vi "Firmware.vi"() -> ()   [LabVIEW 2017]
uses:
  <vilib>/Platform/TimedLoop/XDataNode/timing_clust.ctl
  <vilib>/Platform/TimedLoop/XDataNode/nitl_modes.ctl
  <vilib>/Platform/TimedLoop/XDataNode/wakeup.ctl
  modInput.ctl
  <instrlib>/_niInstr/Instruction Framework/v1/FPGA/Helper Classes/Single Address Space Collection/Single Address Space Collection.lvclass
  C:/Program Files (x86)/National Instruments/LabVIEW 2017/instr.lib/_niInstr/Instruction Framework/v1/FPGA/Interfaces/Address Space Collection/Address Space Collection.lvclass
  <instrlib>/_niInstr/FIFO Register Bus/v1/FPGA/niInstr FIFO Register Bus v1 FPGA.lvclass
  C:/Program Files (x86)/National Instruments/LabVIEW 2017/instr.lib/_niInstr/Instruction Framework/v1/FPGA/Interfaces/Instruction Producer/Instruction Producer.lvclass
  <vilib>/rvi/Emulation/niFpgaGetClockAttributes.vi
  <vilib>/rvi/Emulation/niFpgaSctlEmulationGetInTimedLoop.vi
  <vilib>/rvi/Emulation/niFpgaEmulationReportErrorSimple.vi
  <vilib>/rvi/Emulation/niFpgaProcessEmulError.vi
  <vilib>/rvi/Emulation/niFpgaCriticalErrorInLSC.vi
  <vilib>/rvi/eio/common/nirviEmuTemplateMethod_errors.vi
  <vilib>/eio/EIONode/EIONode.xnode
  <vilib>/Platform/TimedLoop/XDataNode/XDataNode.xnode
  <instrlib>/_niInstr/Instruction Framework/v1/FPGA/Top Level Bus/Register Configuration/Register Configuration.lvclass
  <vilib>/Platform/TimedLoop/XDataNode/XDNodeRunTimeDep.lvlib
  <vilib>/NI/PowerElectronicsControl/ScaleAndLimit/Core/ScaleAndLimit.lvlib
  <vilib>/NI/PowerElectronicsControl/ScaleAndLimit/Core/AddressSpace.lvclass
  <vilib>/NI/PowerElectronicsControl/WaveformAcq/FPGA/WaveformAddressSpace.lvclass
  BuckBoost.lvlib
  AddressSpace.lvclass
panel:
  out "errors":sgl[](array[numeric])
  out "I_BuckBoost":sgl[](array[numeric])
  out "perturbance":sgl
  in  "desiredSimultaneousAILoopRate":u32 caption="Count(Ticks)"
  out "actualBuckBoostRate":u32
  in  "desiredBuckBoostRate":u32
  out "signal":fxp<+,18,0>[](array[numeric])
  in  "I_setpt":sgl format="%#_13g"
  in  "ManualTrigger":bool
  out "TriggerTimestamp":i32
  out "FaultBuffer":u64 format="%.0x"
  out "relativeTimestamp":i32
  in  "fifo reg bus ctrl 0":u32
  out "fifo reg bus status 0":u32
  out "fifo reg bus data 0":u64
  out "actualSimultaneousAILoopRate":u32
  out "LimitsFlag":bool
  out "Simultaneous_AI":sgl[](array[numeric])
  # "Device Utilization\n---------------------------\nTotal Slices: 66.8% (8878 out of 13300)\nSlice Registers: 25.5% (27136 out of 106400)\nSlice LUTs: 44.1% (23463 out of 53200)\nBlock RAMs: 5.0% (7 out of 140)\nDSP48s: 1.8% (4 out of 220)"
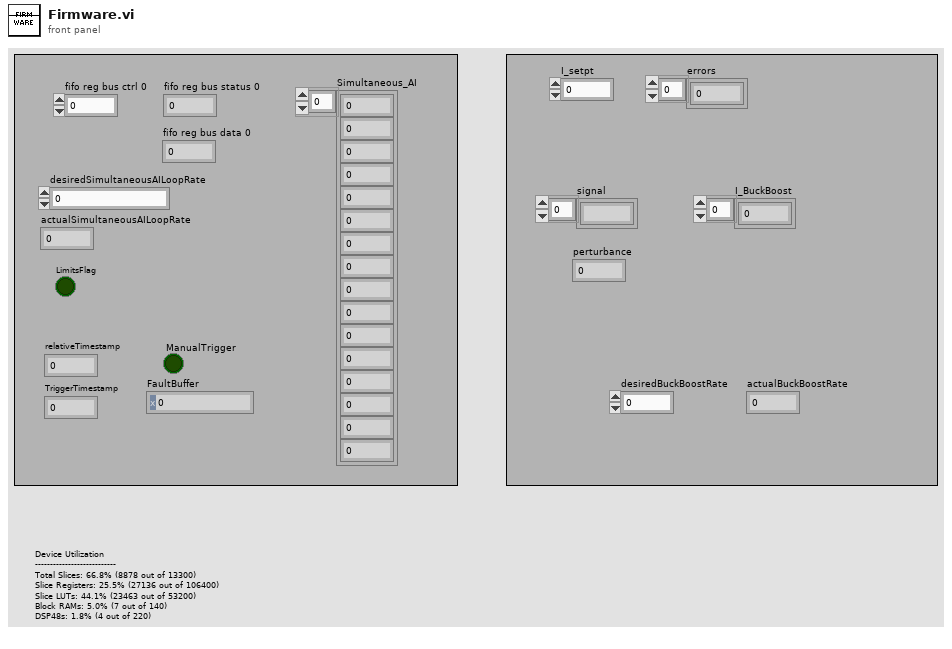
[diagram p1: front panel]
types:
  T1 = typedef "BuckBoost.lvlib/contSettings.ctl" = cluster{"numberOfInterleaves":refnum<k21>, "rampRate":refnum<k21>, "manualInput":refnum<k21>, "perturbAmp":refnum<k21>, "perturbAngleInc":refnum<k21>, "reset":refnum<k21>, "state":refnum<k21>, "gains":refnum<k21>, "Currents":refnum<k21>}
  T2 = typedef "BuckBoost.lvlib/modRegisters.ctl" = cluster{"numberOfInterleaves":refnum<k21>, "Enable":refnum<k21>, "triangleInc":refnum<k21>, "Deadband":refnum<k21>, "Enabled":refnum<k21>}
  T3 = typedef "XDNodeRunTimeDep.lvlib/timing_clust.ctl" = cluster{"Expected End [f-1]":u64, "Actual End [f-1]":u64, "Finished Late? [f-1]":bool, "Expected End [i-1]":u64, "Actual End [i-1]":u64, "Finished Late? [i-1]":bool, "Expected Start [i]":u64, "Actual Start [i]":u64, "Expected Start [f]":u64, "Actual Start [f]":u64, "Source Name":string, "Structure Name":string, "Period":i64, "Deadline":i64, "Offset":i64, "Start":i64, "Priority":i32, "Timeout":i32, "Mode":T4, "Wakeup Reason":T5, "Error":errorcluster, "Source Type":string, "Secondary Source Type":string, "Global End Time":u64, "Global Start Time":u64, "Frame Duration":u64, "Iteration Duration":u64, "Assigned CPU":i32, "I/O Scan Engine Mode":u32}
  T4 = typedef "XDNodeRunTimeDep.lvlib/nitl_modes.ctl" = enum32{"No Change", "Process missed periods, maintain original phase", "Discard missed periods, maintain original phase", "Process missed periods, ignore original phase", "Discard missed periods, ignore original phase"}
  T5 = typedef "XDNodeRunTimeDep.lvlib/wakeup.ctl" = enum32{"Normal", "Aborted", "Asynchronous wakeup", "Timing source error", "Timed loop error", "Timeout"}
  T6 = typedef "BuckBoost.lvlib/modInput.ctl" = cluster{"signal":fxp<+,18,0>[]}
  T7 = typedef "BuckBoost.lvlib/modOutput.ctl" = cluster{"Top":bool, "Bottom":bool}
  T8 = typedef "ScaleAndLimit.lvlib/LimitsRegisters.ctl" = cluster{"HighLimits":refnum<k21>, "LowLimits":refnum<k21>, "ClearLimits":refnum<k21>, "LimitsFlag":refnum<k21>}
  T9 = typedef "ScaleAndLimit.lvlib/ConfigRegisters.ctl" = cluster{"LimitsEnabled":refnum<k21>, "UnscaledHighLimit":refnum<k21>, "UnscaledLowLimit":refnum<k21>, "B":refnum<k21>, "M":refnum<k21>}
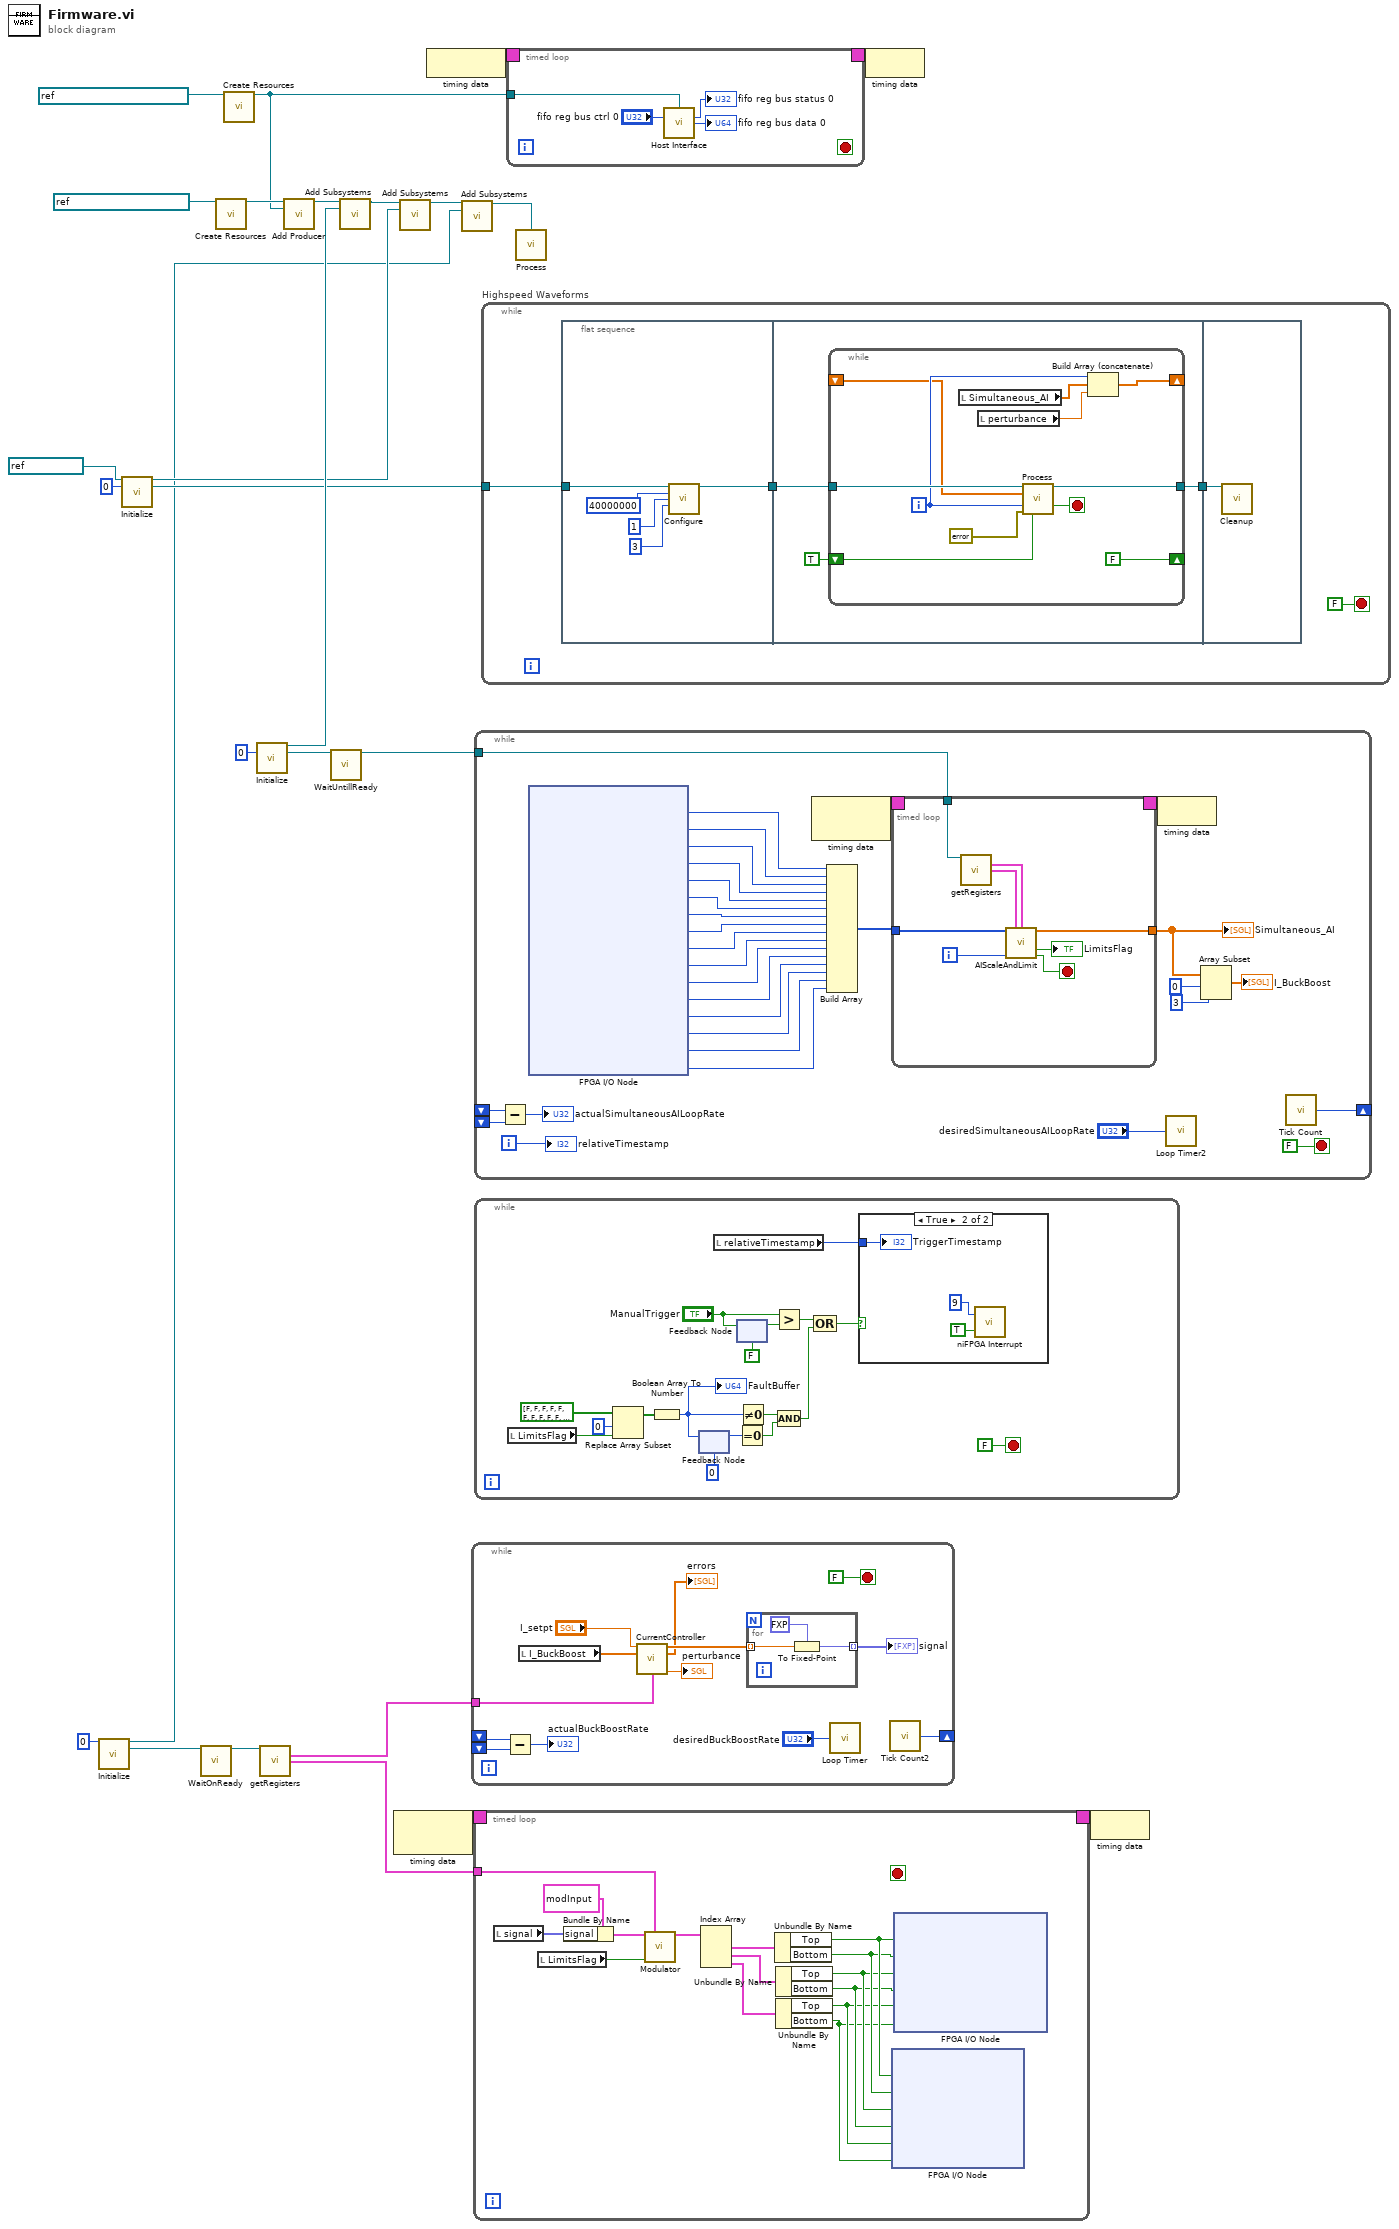
[diagram p0: block diagram]
diagram:
  n1 = call <vilib>:"Initialize.vi"("instance"=u8 0) -> ("subsystem"=w9:refnum<class "Single Address Space Collection.lvclass">, "AddressSpace"=w6:refnum<class "AddressSpace.lvclass">)  [unwired: 13 in]
  n2 = call <vilib>:"Initialize.vi"("DMA FIFO"=refnum<k21> "DataSGL0" ("FIFO Out"), "instance"=u8 0) -> ("subsystem"=w12:refnum<class "Single Address Space Collection.lvclass">, "AddressSpace"=w15:refnum<class "WaveformAddressSpace.lvclass">)  [unwired: 12 in]
  n3 = call "WaitOnReady.vi"("AddressSpace in"=w6) -> ("AddressSpace out"=w5:refnum<class "AddressSpace.lvclass">)  [unwired: 14 in]
  n4 = call <instrlib>:"Create Resources.vi"("register clock"=refnum<k21> "40 MHz Onboard Clock") -> ("register configuration"=w24:refnum<class "Register Configuration.lvclass">)  [unwired: 14 in]
  n5 = call <instrlib>:"Create Resources.vi"("instruction fifo"=refnum<k21> "reg.host instruction fifo 0") -> ("fifo register bus"=w16:refnum<class "niInstr FIFO Register Bus v1 FPGA.lvclass">)  [unwired: 14 in]
  n6 = call <vilib>:"Initialize.vi"("instance"=u8 0) -> ("subsystem"=w21:refnum<class "Single Address Space Collection.lvclass">, "AddressSpace"=w19:refnum<class "AddressSpace.lvclass">)  [unwired: 13 in]
  n7 = call <vilib>:"getRegisters.vi"("AddressSpace in"=w5) -> ("settingsReg"=w4:T1, "modRegisters"=w3:T2)  [unwired: 12 in, 1 out]
  n8 = call <instrlib>:"Add Producer.vi"("register configuration in"=w24, "instruction producer"=w16) -> ("register configuration out"=w22:refnum<class "Register Configuration.lvclass">)  [unwired: 13 in]
  n9 = call <vilib>:"WaitUntillReady.vi"("AddressSpace in"=w19) -> ("AddressSpace out"=w18:refnum<class "AddressSpace.lvclass">)  [unwired: 14 in]
  n10 = call <instrlib>:"Add Subsystems.vi"("register configuration in"=w22, "subsystems"=w21) -> ("register configuration out"=w11:refnum<class "Register Configuration.lvclass">)  [unwired: 13 in]
  n11 = node-c288() -> (w8:T3)  [unwired: 1 in]
  n12 = call <instrlib>:"Add Subsystems.vi"("register configuration in"=w11, "subsystems"=w12) -> ("register configuration out"=w10:refnum<class "Register Configuration.lvclass">)  [unwired: 13 in]
  n13 = node-c288() -> (w26:T3)
  n14 = call <instrlib>:"Add Subsystems.vi"("register configuration in"=w10, "subsystems"=w9) -> ("register configuration out"=w1:refnum<class "Register Configuration.lvclass">)  [unwired: 13 in]
  n15 = while {
    shift-right: [w35] -> _
    shift-left: _ -> [w33]
    shift-left: _ -> [w34]
    tunnel: w4 -> [w30]
    stop <- FALSE stop-if-true
    n16 = Subtract(x=w33, y=w34) -> (x-y=→"actualBuckBoostRate":u32)
    n17 = local read "I_BuckBoost"() -> (w28:sgl[])
    n18 = call "CurrentController.vi"("I_setpt"="I_setpt", "I_procVar"=w28, "settings"=w30) -> ("output"=w39:sgl[], "errors"=→"errors":sgl[], "perturbance"=→"perturbance":sgl)  [unwired: 10 in]
    n19 = for {
      tunnel: w39 -> [w40] mode=indexing
      tunnel: [w41] -> w37 mode=indexing
      n20 = To Fixed-Point(fixed-point type=fxp<+,18,0> 0.0 ("triangle"), number=w40) -> (fixed-point=w41:fxp<+,18,0>)
    }
    "signal" <- w37
    n21 = call "Loop Timer"("Count(Ticks)"="desiredBuckBoostRate") -> ()  [unwired: 1 out]
    n22 = call "Tick Count2"() -> ("Tick Count(Ticks)"=w35:u32)
  }
  n23 = timed-loop {
    timing: w8 -> [_]
    timing-out: [_] -> w7
    tunnel: w3 -> [w55]
    stop <- _ stop-if-true
    n24 = local read "signal"() -> (w53:fxp<+,18,0>[])
    n25 = local read "LimitsFlag"() -> (w54:bool)
    n26 = Bundle By Name(cluster=T6 {"signal"=[0.0, 0.0, 0.0, 0.0]} ("input"), "signal"=w53) -> (w56:T6)
    n27 = call "Modulator.vi"("input"=w56, "modRegisters"=w55, "Disable"=w54) -> ("output"=w52:T7[])  [unwired: 12 in]
    n28 = Index Array(array=w52) -> (element #1=w51:T7, element #2=w50:T7, element #3=w49:T7)  [unwired: 3 in]
    n29 = Unbundle By Name(w51) -> ("Top"=w48:bool, "Bottom"=w47:bool)
    n30 = Unbundle By Name(w50) -> ("Top"=w46:bool, "Bottom"=w45:bool)
    n31 = Unbundle By Name(w49) -> ("Top"=w44:bool, "Bottom"=w43:bool)
    n32 = xnode "FPGA I/O Node"("RMC/LVTTL/DIO6"=w48, "RMC/LVTTL/DIO7"=w47, "RMC/LVTTL/DIO8"=w46, "RMC/LVTTL/DIO9"=w45, "RMC/LVTTL/DIO10"=w44, "RMC/LVTTL/DIO11"=w43) -> ()  [unwired: 6 in, 6 out]
    n33 = xnode "FPGA I/O Node"("RMC/Half-Bridge/DO6"=w48, "RMC/Half-Bridge/DO7"=w47, "RMC/Half-Bridge/DO8"=w46, "RMC/Half-Bridge/DO9"=w45, "RMC/Half-Bridge/DO10"=w44, "RMC/Half-Bridge/DO11"=w43) -> ()  [unwired: 6 in, 6 out]
  }
  n34 = while {
    shift-right: [w89] -> _
    shift-left: _ -> [w88]
    shift-left: _ -> [w87]
    tunnel: w18 -> [w68]
    i -> [w65]
    stop <- FALSE stop-if-true
    n35 = Subtract(x=w88, y=w87) -> (x-y=→"actualSimultaneousAILoopRate":u32)
    n36 = xnode "FPGA I/O Node"() -> ("RMC/Simultaneous/AI0"=w85:i16, "RMC/Simultaneous/AI1"=w84:i16, "RMC/Simultaneous/AI2"=w83:i16, "RMC/Simultaneous/AI3"=w82:i16, "RMC/Simultaneous/AI4"=w81:i16, "RMC/Simultaneous/AI5"=w80:i16, "RMC/Simultaneous/AI6"=w79:i16, "RMC/Simultaneous/AI7"=w78:i16, "RMC/Simultaneous/AI8"=w77:i16, "RMC/Simultaneous/AI9"=w76:i16, "RMC/Simultaneous/AI10"=w75:i16, "RMC/Simultaneous/AI11"=w74:i16, "RMC/Simultaneous/AI12"=w73:i16, "RMC/Simultaneous/AI13"=w72:i16, "RMC/Simultaneous/AI14"=w71:i16, "RMC/Simultaneous/AI15"=w66:i16)  [unwired: 16 in, 16 out]
    n37 = node-c288() -> (w70:T3)  [unwired: 1 in]
    n38 = Build Array(w85, w84, w83, w82, w81, w80, w79, w78, w77, w76, w75, w74, w73, w72, w71, w66) -> (w67:i16[])
    n39 = timed-loop {
      timing: w70 -> [_]
      timing-out: [_] -> w69
      tunnel: w67 -> [w98]
      tunnel: [w97] -> w63
      tunnel: w68 -> [w95]
      i -> [w92]
      stop <- w96 stop-if-true
      n40 = call <vilib>:"getRegisters.vi"("AddressSpace in"=w95) -> ("LimitsRegisters"=w93:T8, "ConfigRegisters"=w94:T9)  [unwired: 12 in, 1 out]
      n41 = call <vilib>:"AIScaleAndLimit.vi"("UnscaledAI"=w98, "ConfigRegisters"=w94, "LimitsRegisters"=w93, "index"=w92) -> ("ScaledAI"=w97:sgl[], "Limited"=→"LimitsFlag":bool, "output valid"=w96:bool)  [unwired: 9 in]
    }
    "Simultaneous_AI" <- w63
    n42 = node-c288(w69) -> ()
    n43 = call "Loop Timer2"("Count(Ticks)"="desiredSimultaneousAILoopRate") -> ()  [unwired: 1 out]
    n44 = Array Subset(array=w63, index=0, length=3) -> (→"I_BuckBoost":sgl[])
    n45 = call "Tick Count"() -> ("Tick Count(Ticks)"=w89:u32)
    "relativeTimestamp" <- w65
  }
  n46 = while {
    stop <- FALSE stop-if-true
    n47 = local read "LimitsFlag"() -> (w111:bool)
    n48 = Replace Array Subset(array=bool[] [FALSE, FALSE, FALSE, FALSE, FALSE, FALSE, FALSE, FALSE, FALSE, FALSE, FALSE, FALSE, FALSE, FALSE, FALSE, FALSE, FALSE, FALSE, FALSE, FALSE, FALSE, FALSE, FALSE, FALSE, FALSE, FALSE, FALSE, FALSE, FALSE, FALSE, FALSE, FALSE, FALSE, FALSE, FALSE, FALSE, FALSE, FALSE, FALSE, FALSE, FALSE, FALSE, FALSE, FALSE, FALSE, FALSE, FALSE, FALSE, FALSE, FALSE, FALSE, FALSE, FALSE, FALSE, FALSE, FALSE, FALSE, FALSE, FALSE, FALSE, FALSE, FALSE, FALSE, FALSE], new element=w111, index=0) -> (w109:bool[])
    n49 = Boolean Array To Number(Boolean array=w109) -> (number=w107:u64)
    "FaultBuffer" <- w107
    n50 = feedback-in #1(w107) -> ()
    n51 = feedback #1(u64 0) -> (w106:u64)
    n52 = local read "relativeTimestamp"() -> (w113:i32)
    n53 = feedback-in #2("ManualTrigger") -> ()
    n54 = feedback #2(FALSE ("ManualTrigger")) -> (w117:bool)
    n55 = Equal To 0?(x=w106) -> (x = 0?=w104:bool)
    n56 = Not Equal To 0?(x=w107) -> (x != 0?=w105:bool)
    n57 = Greater?(x="ManualTrigger", y=w117) -> (0:w118:bool)
    n58 = Compound Arithmetic op=AND(w105, w104) -> (w103:bool)
    n59 = Compound Arithmetic op=OR(w118, w103) -> (w115:bool)
    n60 = case shown="True" w115 {
      tunnel: w113 -> [_ w120]
      frame False {
      }
      frame True {
        n61 = call <vilib>:"niFPGA Interrupt.vi"("Wait Until Cleared (F)"=TRUE, "IRQ Number (0)"=u8 9) -> ()  [unwired: 1 in]
        "TriggerTimestamp" <- w120
      }
    }
  }
  n62 = while "Highspeed Waveforms" {
    tunnel: w15 -> [w123]
    stop <- FALSE stop-if-true
    n63 = flat-sequence {
      tunnel: [w127] -> w125
      tunnel: w123 -> [w128]
      tunnel: w125 -> [w134]
      tunnel: [w133] -> w124
      tunnel: w124 -> [w146]
      frame #0 {
        n64 = call <vilib>:"Configure.vi"("WaveformAddressSpace in"=w128, "oclk_freq"=u32 40000000, "oclk_mult"=u32 1, "UnderflowMargin"=u32 3 ("y")) -> ("WaveformAddressSpace out"=w127:refnum<class "WaveformAddressSpace.lvclass">)  [unwired: 11 in]
      }
      frame #1 {
        n65 = while {
          shift-right: [w144] -> _
          shift-left: _ -> [w136]
          shift-right: [FALSE] -> _
          shift-left: TRUE -> [w139]
          tunnel: w134 -> [w141]
          tunnel: [w140] -> w133
          i -> [w138]
          stop <- w142 stop-if-true
          n66 = local read "Simultaneous_AI"() -> (w137:sgl[])
          n67 = local read "perturbance"() -> (w135:sgl)
          n68 = call <instrlib>:"Process.vi"("WaveformAddressSpace in"=w141, "Data"=w136, "Iteration"=w138, "error in (no error)"=errorcluster {"status"=FALSE, "code"=0, "source"=""} ("injectError1"), "FirstIteration"=w139) -> ("WaveformAddressSpace out"=w140:refnum<class "WaveformAddressSpace.lvclass">, "stop"=w142:bool)  [unwired: 7 in, 2 out]
          n69 = Build Array (concatenate)(w138, w137, w135) -> (w144:sgl[])
        }
      }
      frame #2 {
        n70 = call <vilib>:"Cleanup.vi"("WaveformAddressSpace in"=w146) -> ()  [unwired: 14 in, 1 out]
      }
    }
  }
  n71 = timed-loop {
    timing: w26 -> [_]
    timing-out: [_] -> w25
    tunnel: w16 -> [w150]
    stop <- _ stop-if-true
    n72 = call <instrlib>:"Host Interface.vi"("fifo register bus"=w150, "fifo reg bus ctrl 0"="fifo reg bus ctrl 0") -> ("fifo reg bus status 0"=→"fifo reg bus status 0":u32, "fifo reg bus data 0"=→"fifo reg bus data 0":u64)  [unwired: 12 in]
  }
  n73 = call <instrlib>:"Process.vi"("register configuration"=w1) -> ()  [unwired: 15 in]
  n74 = node-c288(w25) -> ()
  n75 = node-c288(w7) -> ()
